vi "start_scope.vi"(0 "resource name":refnum<k15>, 1 "Controls cluster":T5 {"C1 vertical coupling / V" items=["AC", "DC", "Ground"]; "C2 vertical coupling / V" items=["AC", "DC", "Ground"]; "Trigger slope" items=["Positive", "Negative"]}, 5 "Current VI's Path":path=path "" caption="start path", 9 "Load old conditions":bool, 11 "error in":errorcluster, 12 "Controls References Cluster In":T1) -> (3 "Controls cluster out":T5 {"C1 vertical coupling / V" items=["AC", "DC", "Ground"]; "C2 vertical coupling / V" items=["AC", "DC", "Ground"]; "Trigger slope" items=["Positive", "Negative"]}, 4 "instrument handle out":refnum<k15>, 14 "Controls References Cluster Out":T1, 15 "error out":errorcluster)   [LabVIEW 2023]
uses:
  <instrlib>/niScope/Controls/niScope trigger slope.ctl
  <instrlib>/niScope/Controls/niScope trigger source.ctl
  <instrlib>/niScope/Controls/niScope vertical coupling.ctl
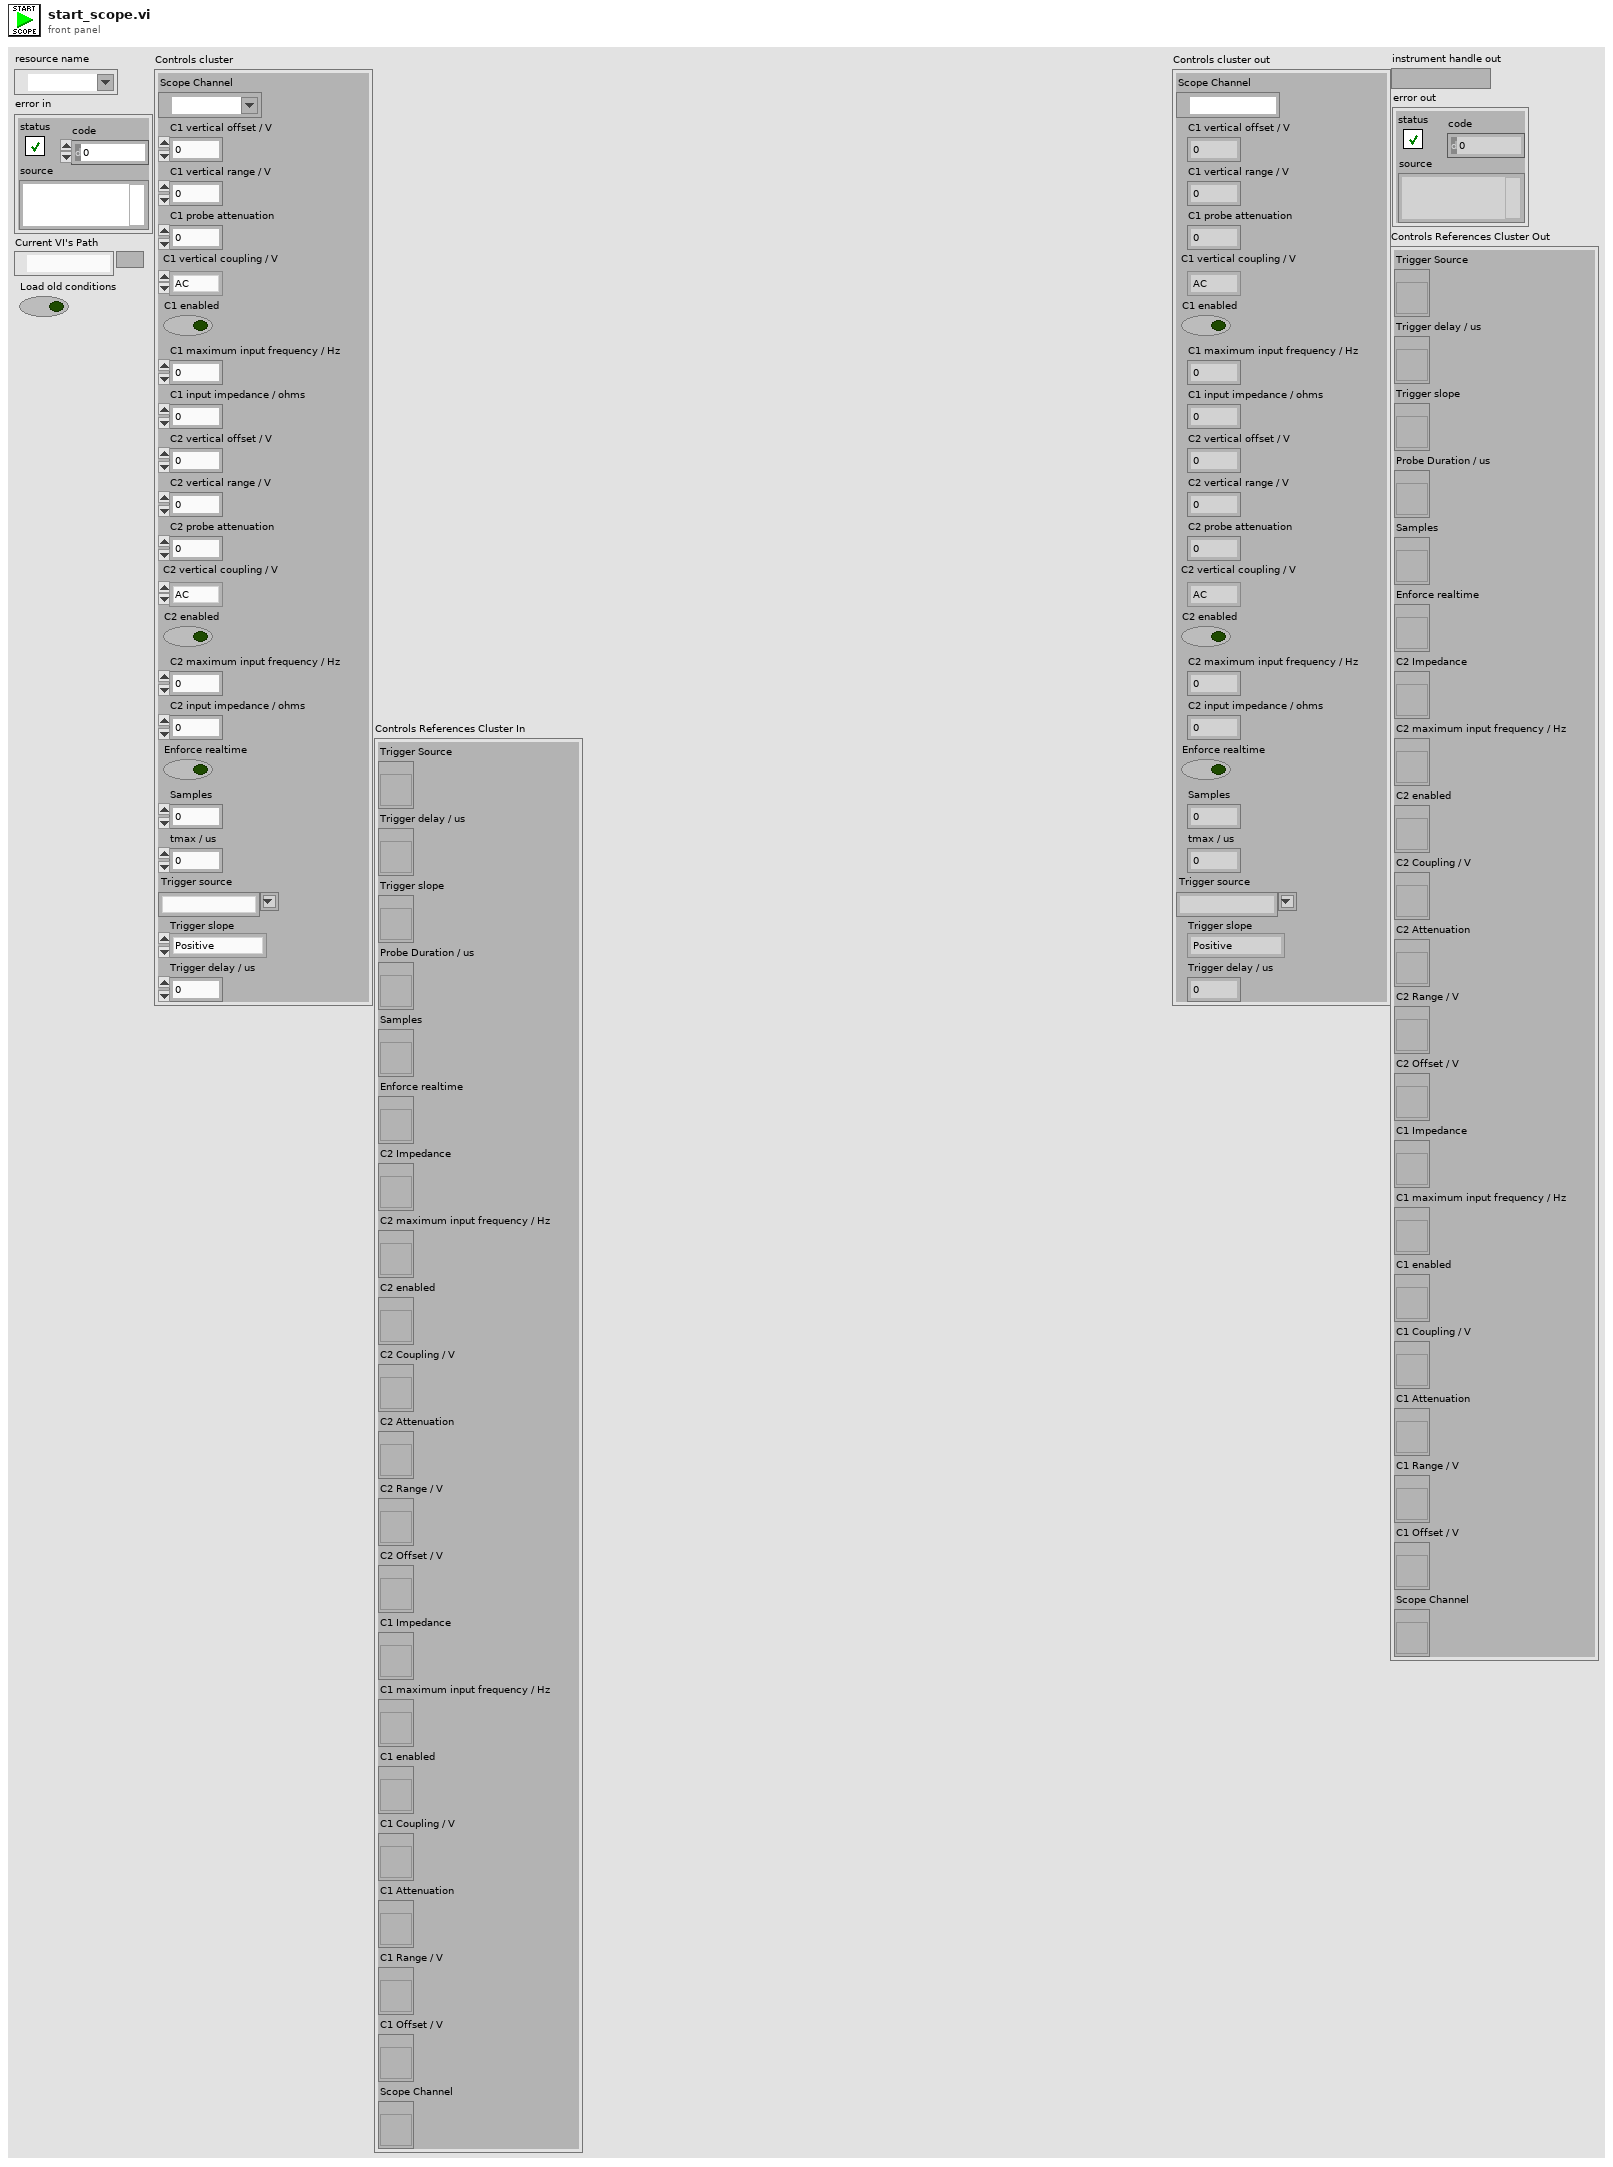
[diagram p1: front panel]
types:
  T1 = cluster{"Trigger Source":refnum<vi>, "Trigger delay / us":refnum<vi>, "Trigger slope":refnum<vi>, "Probe Duration / us":refnum<vi>, "Samples":refnum<vi>, "Enforce realtime":refnum<vi>, "C2 Impedance":refnum<vi>, "C2 maximum input frequency / Hz":refnum<vi>, "C2 enabled":refnum<vi>, "C2 Coupling / V":refnum<vi>, "C2 Attenuation":refnum<vi>, "C2 Range / V":refnum<vi>, "C2 Offset / V":refnum<vi>, "C1 Impedance":refnum<vi>, "C1 maximum input frequency / Hz":refnum<vi>, "C1 enabled":refnum<vi>, "C1 Coupling / V":refnum<vi>, "C1 Attenuation":refnum<vi>, "C1 Range / V":refnum<vi>, "C1 Offset / V":refnum<vi>, "Scope Channel":refnum<vi>}
  T2 = typedef "niScope vertical coupling.ctl" = i32
  T3 = typedef "niScope trigger source.ctl" = string
  T4 = typedef "niScope trigger slope.ctl" = i32
  T5 = cluster{"Scope Channel":refnum<k15>, "C1 vertical offset / V":dbl, "C1 vertical range / V":dbl, "C1 probe attenuation":dbl, "C1 vertical coupling / V":T2, "C1 enabled":bool, "C1 maximum input frequency / Hz":dbl, "C1 input impedance / ohms":u32, "C2 vertical offset / V":dbl, "C2 vertical range / V":dbl, "C2 probe attenuation":dbl, "C2 vertical coupling / V":T2, "C2 enabled":bool, "C2 maximum input frequency / Hz":dbl, "C2 input impedance / ohms":u32, "Enforce realtime":bool, "Samples":i64, "tmax / us ":dbl, "Trigger source":T3, "Trigger slope":T4, "Trigger delay / us":dbl}
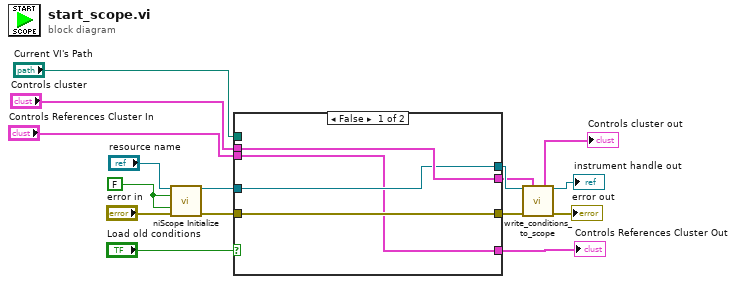
[diagram p0: block diagram]
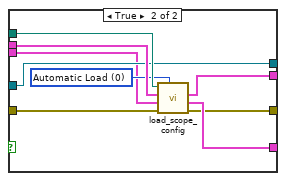
[diagram p2: hidden frame]
diagram:
  w14 = FALSE ("id query")
  n1 = call <instrlib>:"niScope Initialize.vi"("resource name"="resource name", "id query"=w14, "reset device"=w14, "error in"="error in") -> ("instrument handle"=w13:refnum<k15>, "error out"=w12:errorcluster)  [unwired: 10 in]
  n2 = case shown="False" "Load old conditions" {
    tunnel: w13 -> [w18 w23]
    tunnel: w12 -> [w19 w29]
    tunnel: "Controls cluster" -> [w20 w28]
    tunnel: [w17 w27] -> w2
    tunnel: [w20 w26] -> w6
    tunnel: [w19 w25] -> w8
    tunnel: "Current VI's Path" -> [_ w24]
    tunnel: [w18 w23] -> w7
    tunnel: "Controls References Cluster In" -> [w17 w21]
    frame False {
    }
    frame True {
      w22 = u16 0 items=["Automatic Load", "Custom File"] ("Load File Type")
      n3 = call "load_scope_config.vi"("Load File Type"=w22, "error in"=w29, "Controls References Cluster In"=w21, "Controls cluster"=w28, "Current VI's Path"=w24) -> ("error out"=w25:errorcluster, "Controls References Cluster Out"=w27:T1, "Controls cluster out"=w26:T5)  [unwired: 4 in]
    }
  }
  "Controls References Cluster Out" <- w2
  n4 = call "write_conditions_to_scope.vi"("instrument handle"=w7, "Controls Cluster In"=w6, "error in"=w8) -> ("Controls Cluster Out"=→"Controls cluster out":T5, "instrument handle out"=→"instrument handle out":refnum<k15>, "error out"=→"error out":errorcluster)  [unwired: 10 in]
